vi "host_initialize.vi"(8 "error in":errorcluster) -> (0 "error out":errorcluster)   [LabVIEW 2021]
uses:
  host_global_vars.vi
  <vilib>/FPGAPlugInAG/PXIe-7856R/niLvFpga_Open_PXIe-7856R.vi
  <vilib>/rvi/interface/nirviOpenFPGA/nirviOpenFPGA.xnode
  FPGA Bitfiles/openlabspm_FPGATarget_fpgamain_eo-gUZR5D1g.lvbitx
  fpga/fpga_main.vi
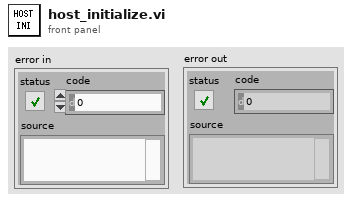
[diagram p1: front panel]
types:
  T1 = enum16{"open", "replace", "create", "open or create", "replace or create", "replace or create with confirmation"}
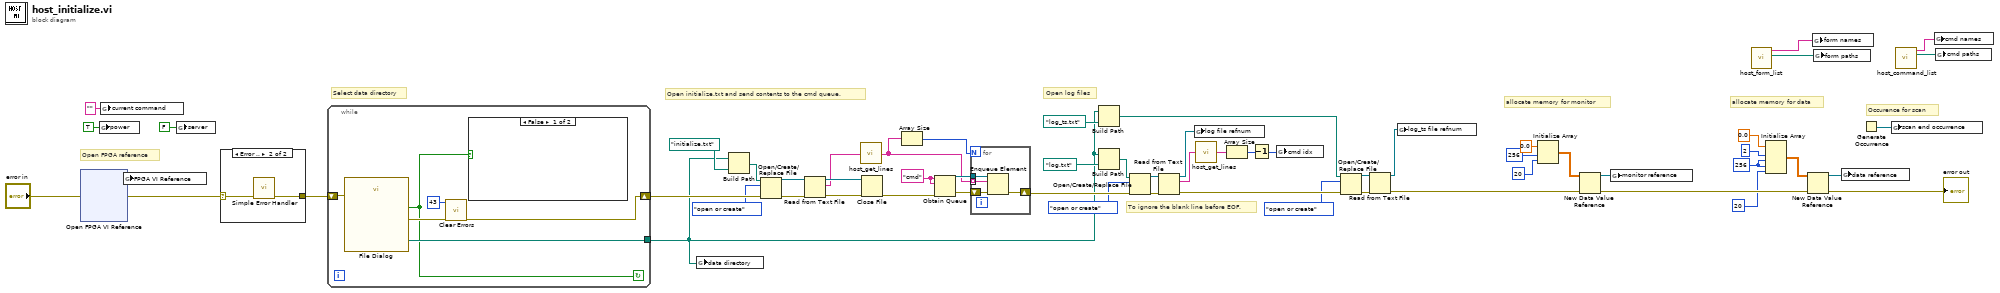
[diagram p0: block diagram]
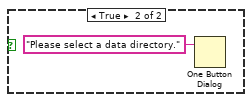
[diagram p3: hidden frame]
diagram:
  w17 = 256 ("dimension size")
  w49 = "cmd" ("name (unnamed)")
  # "Occurence for scan"
  # "allocate memory for data"
  # "To ignore the blank line before EOF."
  # "Open log files"
  # "allocate memory for monitor"
  # "Select data directory"
  # "Open initialize.txt and send contents to the cmd queue."
  # "Open FPGA reference"
  n1 = xnode "Open FPGA VI Reference"("error in"="error in") -> ("FPGA VI Reference Out"=w59:refnum<k20>, "error out"=w2:errorcluster)  [unwired: 1 in]
  n2 = global write "host_global_vars.vi" "power"(TRUE ("power")) -> ()
  n3 = global write "host_global_vars.vi" "current command"("" ("current command")) -> ()
  n4 = global write "host_global_vars.vi" "FPGA VI Reference"(w59) -> ()
  n5 = global write "host_global_vars.vi" "server"(FALSE ("power")) -> ()
  n6 = case shown="Error .." w2 {
    selector: w2 -> [w61 w63]
    tunnel: [w61 w62] -> w1
    frame No Error {
    }
    frame Error {
      n7 = call <vilib>:"Simple Error Handler.vi"("error in (no error)"=w63) -> ("error out"=w62:errorcluster)  [unwired: 4 in, 4 out]
    }
  }
  n8 = while {
    tunnel: [w68] -> w10
    shift-right: [w64] -> w50
    shift-left: w1 -> [w69]
    stop <- w65 continue-if-true
    n9 = call "File Dialog"("error in"=w69) -> ("selected path"=w68:path, "cancelled"=w65:bool, "error out"=w67:errorcluster)  [unwired: 11 in, 1 out]
    n10 = call <vilib>:"Clear Errors.vi"("error in (no error)"=w67, "specific error code to clear (0: all)"=43) -> ("error out"=w64:errorcluster)  [unwired: 4 in, 1 out]
    n11 = case shown="False" w65 {
      frame False {
      }
      frame True {
        n12 = One Button Dialog(message="Please select a data directory.") -> ()  [unwired: 1 in, 1 out]
      }
    }
  }
  n13 = global write "host_global_vars.vi" "data directory"(w10) -> ()
  n14 = Build Path(base path=w10, name or relative path=path "initialize.txt") -> (appended path=w56:path)
  n15 = Open/Create/Replace File(file path (use dialog)=w56, error in=w50, operation (0:open)=T1."open or create") -> (refnum out=w55:refnum<file>, error out=w54:errorcluster)  [unwired: 3 in, 1 out]
  n16 = Read from Text File(file (use dialog)=w55, error in=w54) -> (refnum out=w52:refnum<file>, text=w48:string, error out=w53:errorcluster)  [unwired: 2 in, 1 out]
  n17 = call "host_get_lines.vi"("in"=w48) -> ("out"=w14:string[])
  n18 = Close File(refnum=w52, error in=w53) -> (error out=w51:errorcluster)  [unwired: 1 out]
  n19 = Array Size(array=w14) -> (size(s)=w9:i32)
  n20 = Obtain Queue(name (unnamed)=w49, element data type=w49, error in (no error)=w51) -> (queue out=w46:refnum<queue>, error out=w47:errorcluster)  [unwired: 2 in, 1 out]
  n21 = for {
    N: w9 -> [_]
    tunnel: w46 -> [w73]
    tunnel: w14 -> [w72] mode=indexing
    shift-right: [w71] -> w39
    shift-left: w47 -> [w74]
    n22 = Enqueue Element(queue=w73, element=w72, error in (no error)=w74) -> (error out=w71:errorcluster)  [unwired: 1 in, 2 out]
  }
  n23 = Build Path(base path=w10, name or relative path=path "log_ts.txt") -> (appended path=w31:path)
  n24 = Build Path(base path=w10, name or relative path=path "log.txt") -> (appended path=w40:path)
  n25 = Open/Create/Replace File(file path (use dialog)=w40, error in=w39, operation (0:open)=T1."open or create") -> (refnum out=w37:refnum<file>, error out=w38:errorcluster)  [unwired: 3 in, 1 out]
  n26 = Read from Text File(file (use dialog)=w37, error in=w38) -> (refnum out=w35:refnum<file>, text=w36:string, error out=w33:errorcluster)  [unwired: 2 in, 1 out]
  n27 = global write "host_global_vars.vi" "log file refnum"(w35) -> ()
  n28 = call "host_get_lines.vi"("in"=w36) -> ("out"=w25:string[])
  n29 = Array Size(array=w25) -> (size(s)=w24:i32)
  n30 = Decrement(x=w24) -> (x-1=w23:i32)
  n31 = global write "host_global_vars.vi" "cmd idx"(w23) -> ()
  n32 = Open/Create/Replace File(file path (use dialog)=w31, error in=w33, operation (0:open)=T1."open or create") -> (refnum out=w26:refnum<file>, error out=w34:errorcluster)  [unwired: 3 in, 1 out]
  n33 = Read from Text File(file (use dialog)=w26, error in=w34) -> (refnum out=w30:refnum<file>, error out=w29:errorcluster)  [unwired: 2 in, 2 out]
  n34 = global write "host_global_vars.vi" "log_ts file refnum"(w30) -> ()
  n35 = Initialize Array(sgl 0.0 ("element"), 256 ("dimension size"), 20 ("dimension size")) -> (w43:sgl[][])
  n36 = New Data Value Reference(data value=w43, error in=w29) -> (data value reference=w13:refnum<data-value>, error out=w19:errorcluster)
  n37 = global write "host_global_vars.vi" "monitor reference"(w13) -> ()
  n38 = call "host_form_list.vi"() -> ("paths"=w7:path[], "names"=w6:string[])  [unwired: 10 in]
  n39 = Initialize Array(sgl 0.0 ("element"), 2 ("dimension size"), w17, w17, 20 ("dimension size")) -> (w20:sgl[][][][])
  n40 = New Data Value Reference(data value=w20, error in=w19) -> (data value reference=w12:refnum<data-value>, error out=→"error out":errorcluster)
  n41 = global write "host_global_vars.vi" "form names"(w6) -> ()
  n42 = global write "host_global_vars.vi" "form paths"(w7) -> ()
  n43 = global write "host_global_vars.vi" "data reference"(w12) -> ()
  n44 = Generate Occurrence() -> (w11:refnum<k4>)
  n45 = global write "host_global_vars.vi" "scan end occurrence"(w11) -> ()
  n46 = call "host_command_list.vi"() -> ("paths"=w5:path[], "names"=w4:string[])  [unwired: 10 in]
  n47 = global write "host_global_vars.vi" "cmd names"(w4) -> ()
  n48 = global write "host_global_vars.vi" "cmd paths"(w5) -> ()
